vi "Make Color Table.vi"(0 "Array":u32[](array[colorbox]), 1 "Size":i32=256) -> (2 "Array R":dbl[](array[numeric]), 3 "Array G":dbl[](array[numeric]), 4 "Array B":dbl[](array[numeric]), 5 "Color Tbl":u32[](array[numeric]))   [LabVIEW 2016]
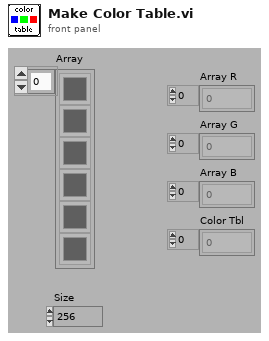
[diagram p1: front panel]
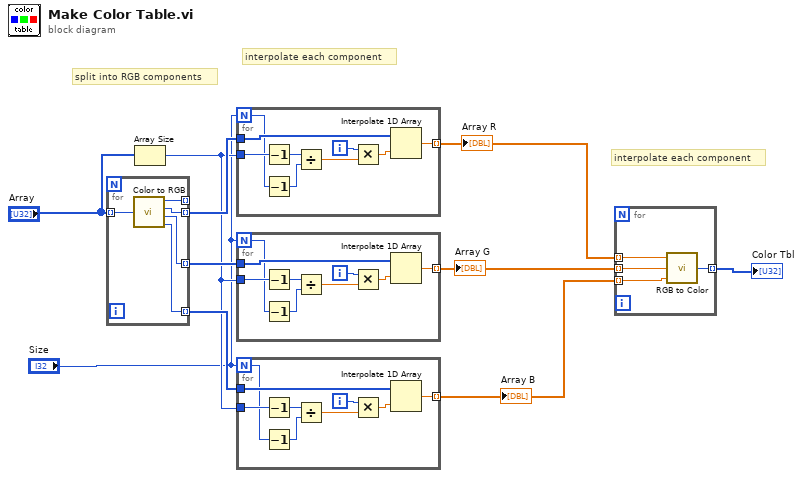
[diagram p0: block diagram]
diagram:
  # "interpolate each component"
  # "interpolate each component"
  # "split into RGB components"
  n1 = for {
    tunnel: "Array" -> [w15] mode=indexing
    tunnel: [w14] -> w9 mode=indexing
    tunnel: [w13] -> w10 mode=indexing
    tunnel: [w12] -> w8 mode=indexing
    tunnel: [w11] -> _ mode=indexing
    n2 = call <vilib>:"Color to RGB.vi"("Color"=w15) -> ("Resolved Color"=w11:u32, "R"=w14:u8, "G"=w13:u8, "B"=w12:u8)
  }
  n3 = Array Size(array="Array") -> (size(s)=w7:i32)
  n4 = for {
    N: "Size" -> [w21]
    tunnel: w9 -> [w24]
    tunnel: [w23] -> w3 mode=indexing
    tunnel: w7 -> [w22]
    i -> [w16]
    n5 = Decrement(x=w22) -> (x-1=w20:i32)
    n6 = Decrement(x=w21) -> (x-1=w19:i32)
    n7 = Divide(x=w20, y=w19) -> (x/y=w17:dbl)
    n8 = Multiply(x=w16, y=w17) -> (x*y=w18:dbl)
    n9 = Interpolate 1D Array(1:w18, 2:w24) -> (0:w23:dbl)
  }
  "Array R" <- w3
  n10 = for {
    N: "Size" -> [w30]
    tunnel: w10 -> [w33]
    tunnel: [w32] -> w4 mode=indexing
    tunnel: w7 -> [w31]
    i -> [w25]
    n11 = Decrement(x=w31) -> (x-1=w29:i32)
    n12 = Decrement(x=w30) -> (x-1=w28:i32)
    n13 = Divide(x=w29, y=w28) -> (x/y=w26:dbl)
    n14 = Multiply(x=w25, y=w26) -> (x*y=w27:dbl)
    n15 = Interpolate 1D Array(1:w27, 2:w33) -> (0:w32:dbl)
  }
  "Array G" <- w4
  n16 = for {
    N: "Size" -> [w39]
    tunnel: w8 -> [w42]
    tunnel: [w41] -> w5 mode=indexing
    tunnel: w7 -> [w40]
    i -> [w34]
    n17 = Decrement(x=w40) -> (x-1=w38:i32)
    n18 = Decrement(x=w39) -> (x-1=w37:i32)
    n19 = Divide(x=w38, y=w37) -> (x/y=w35:dbl)
    n20 = Multiply(x=w34, y=w35) -> (x*y=w36:dbl)
    n21 = Interpolate 1D Array(1:w36, 2:w42) -> (0:w41:dbl)
  }
  "Array B" <- w5
  n22 = for {
    tunnel: w3 -> [w46] mode=indexing
    tunnel: w4 -> [w45] mode=indexing
    tunnel: w5 -> [w44] mode=indexing
    tunnel: [w43] -> w6 mode=indexing
    n23 = call <vilib>:"RGB to Color.vi"("B"=w44, "G"=w45, "R"=w46) -> ("Color"=w43:u32)
  }
  "Color Tbl" <- w6
